vi "Logging Message Loop.vi"(8 "error in (no error)":errorcluster, 10 "Data Queue":refnum<queue>, 11 "Message Queues":T1) -> (0 "error out":errorcluster)   [LabVIEW 2023, in "Logging.lvlib"]
doc: "The message loop subVI to handle messages pertaining to logging data."
uses:
  Logging.lvlib
  support/Message Queue/All Message Queues.ctl
  support/Message Queue/Message Cluster.ctl
  Logging Configuration.ctl
  Logging State.ctl
  support/Message Queue/Enqueue Message (Single).vi
  <vilib>/Utility/error.llb/Error Cluster From Error Code.vi
  <vilib>/ErrorRing/Error Ring.xnode
  support/Message Queue/Message Queue.lvlib
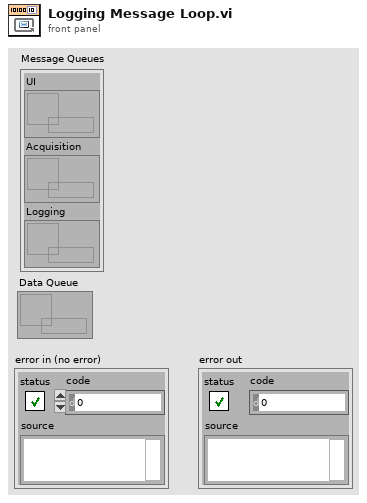
[diagram p1: front panel]
types:
  T1 = typedef "Message Queue.lvlib/All Message Queues.ctl" = cluster{"UI":refnum<queue>, "Acquisition":refnum<queue>, "Logging":refnum<queue>}
  T2 = typedef "Logging.lvlib/Logging Configuration.ctl" = cluster{"Log File Base Path":path, "TDMS File Reference":refnum<k34>}
  T3 = typedef "Logging.lvlib/Logging State.ctl" = enum16{"Idle", "Logging"}
  T4 = enum16{"open", "open or create", "create or replace", "create", "open (read-only)"}
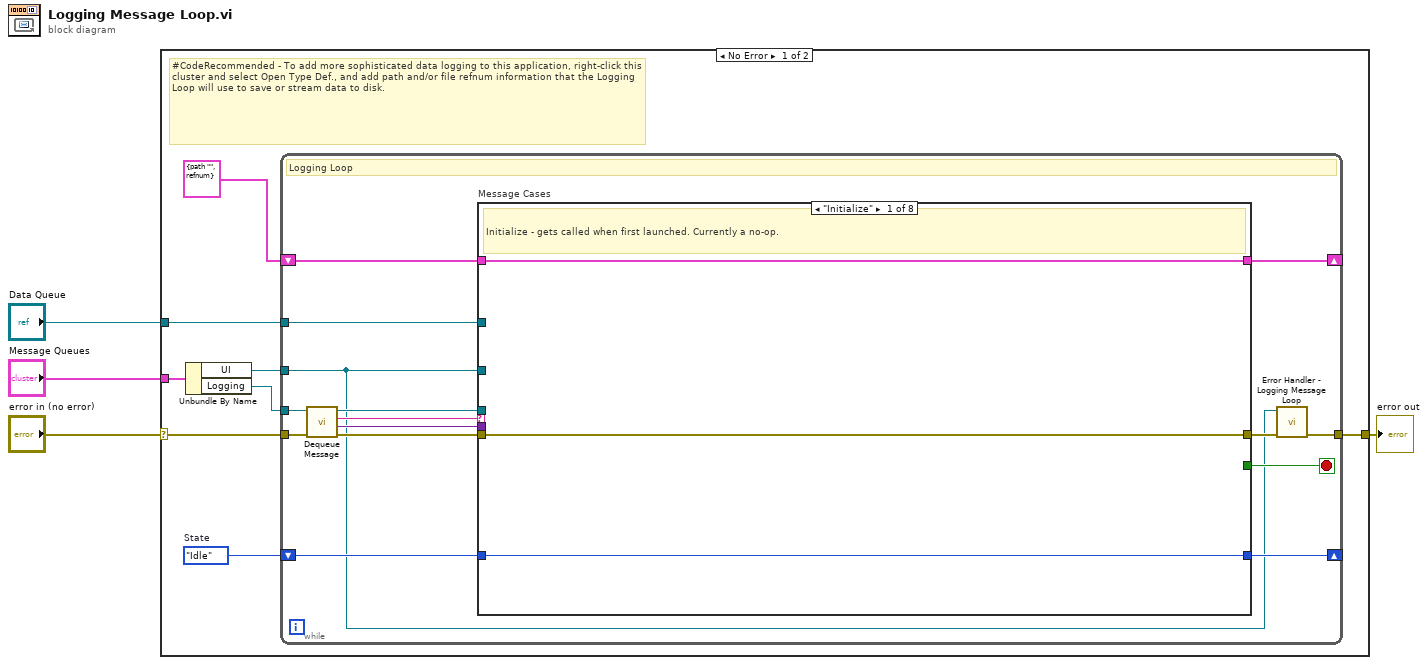
[diagram p0: block diagram]
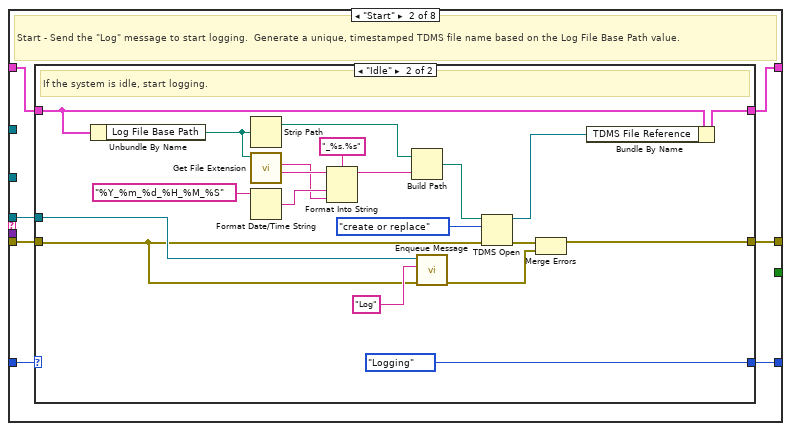
[diagram p2: hidden frame]
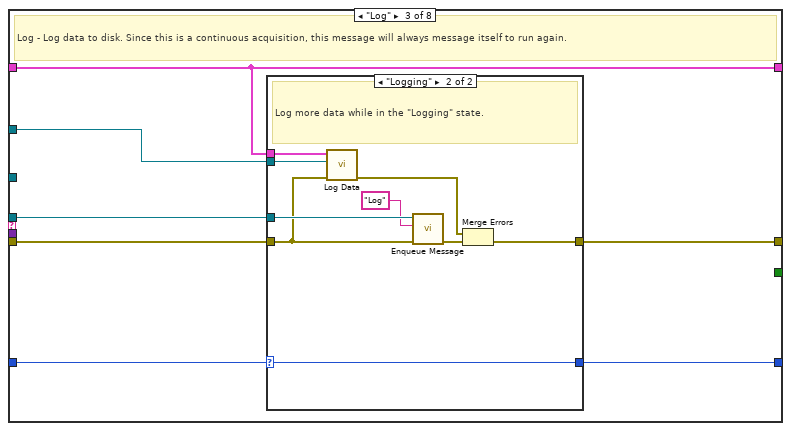
[diagram p4: hidden frame]
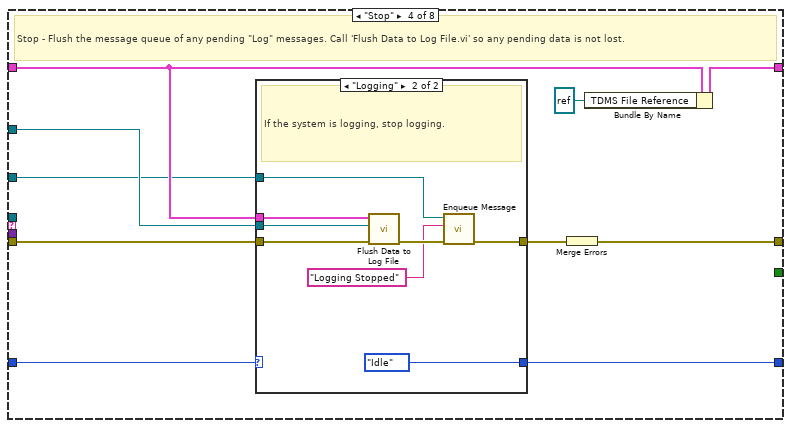
[diagram p6: hidden frame]
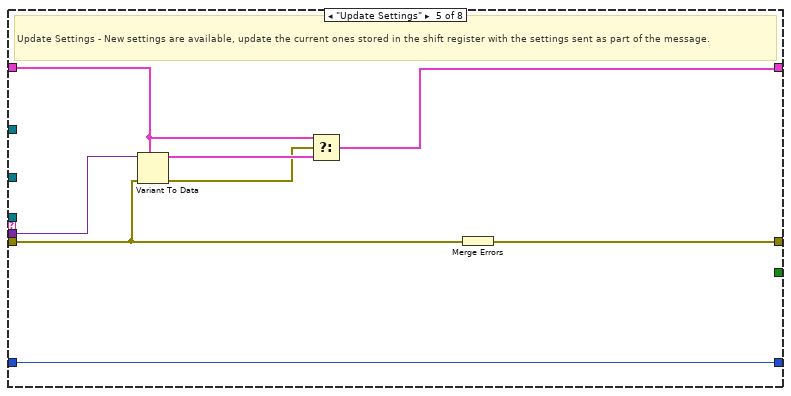
[diagram p8: hidden frame]
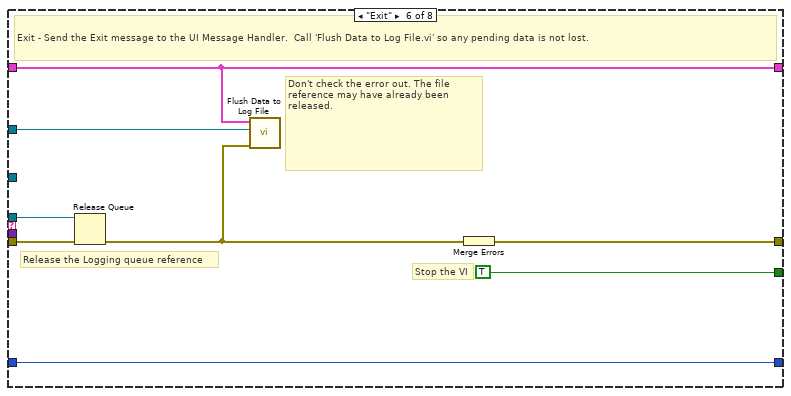
[diagram p9: hidden frame]
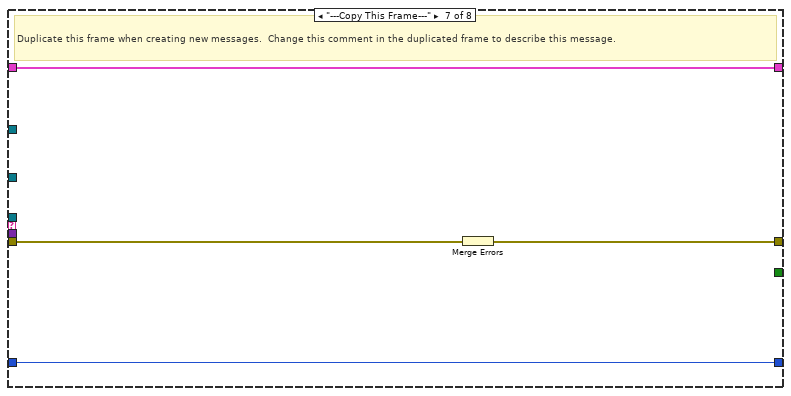
[diagram p10: hidden frame]
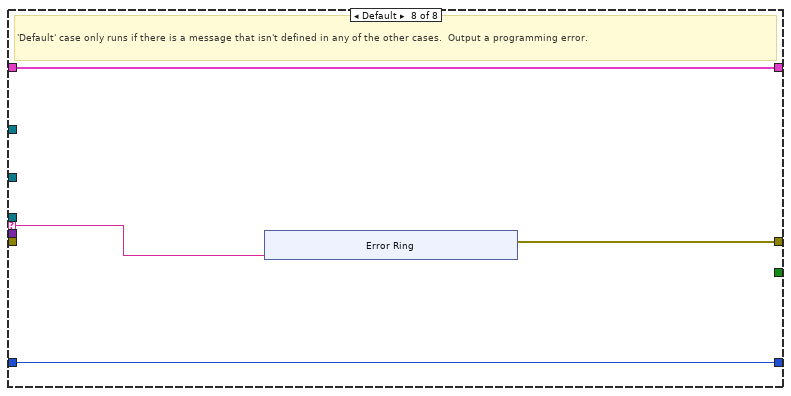
[diagram p11: hidden frame]
diagram:
  n1 = case shown="No Error" "error in (no error)" {
    selector: "error in (no error)" -> [w8 w130]
    tunnel: "Message Queues" -> [w12 _]
    tunnel: [w10 w130] -> w3
    tunnel: "Data Queue" -> [w7 _]
    frame No Error {
      w5 = Logging_State."Idle"  # State
      # "#CodeRecommended - To add more sophisticated data logging to this application, right-click this cluster and select Open Type Def., and add path and/or file refnum information that the Logging Loop will use to save or stream data to disk."
      n2 = Unbundle By Name(w12) -> ("UI"=w6:refnum<queue>, "Logging"=w11:refnum<queue>)
      n3 = while {
        tunnel: w11 -> [w19]
        shift-right: [w26] -> _
        shift-left: T2 {"Log File Base Path"=path "", "TDMS File Reference"=refnum} ("Logging Configuration") -> [w27]
        tunnel: w6 -> [w13]
        tunnel: w7 -> [w18]
        shift-right: [w16] -> _
        shift-left: w5 -> [w17]
        tunnel: w8 -> [w24]
        tunnel: [w15] -> w10
        stop <- w25 stop-if-true
        # "Logging Loop"
        n4 = call "Dequeue Message.vi"("error in (no error)"=w24, "Message Queue"=w19) -> ("error out"=w23:errorcluster, "Message Data"=w21:variant, "Message"=w22:string, "dup Message Queue"=w20:refnum<queue>)  [unwired: 6 in]
        n5 = case "Message Cases" shown="\"Initialize\"" w22 {
          selector: w22 -> [_ _ _ _ _ _ _ w119]
          tunnel: w20 -> [_ w36 w66 _ _ w111 _ _]
          tunnel: w23 -> [w29 w35 w64 w82 w100 w112 w118 _]
          tunnel: [w29 w37 w67 w88 w106 w113 w116 w120] -> w14
          tunnel: w27 -> [w30 w34 w63 w83 w104 w109 w117 w122]
          tunnel: [w30 w33 w63 w86 w101 w109 w117 w122] -> w26
          tunnel: [_ _ _ _ _ TRUE _ _] -> w25
          tunnel: w21 -> [_ _ _ _ w105 _ _ _]
          tunnel: w13 -> [_ _ _ w79 _ _ _ _]
          tunnel: w18 -> [_ _ w65 w84 _ w108 _ _]
          tunnel: w17 -> [w28 w32 w62 w81 w99 w107 w115 w121]
          tunnel: [w28 w31 w61 w80 w99 w107 w115 w121] -> w16
          frame "Initialize" {
            # "Initialize - gets called when first launched. Currently a no-op."
          }
          frame "Start" {
            # "Start - Send the \"Log\" message to start logging.  Generate a unique, timestamped TDMS file name based on the Log File Base Path value."
            n6 = case shown="\"Idle\"" w32 {
              selector: w32 -> [w39 _]
              tunnel: [w38 w42] -> w37
              tunnel: w36 -> [_ w43]
              tunnel: w35 -> [w38 w41]
              tunnel: w34 -> [w40 w44]
              tunnel: [w40 w46] -> w33
              tunnel: [w39 Logging_State."Logging" ("State")] -> w31
              frame "Logging" {
                # "The system is already logging. Ignore the \"Start\" message."
              }
              frame "Idle" {
                # "If the system is idle, start logging."
                n7 = Unbundle By Name(w44) -> ("Log File Base Path"=w59:path)
                n8 = Strip Path(path=w59) -> (stripped path=w56:path)  [unwired: 1 out]
                n9 = call <vilib>:"Get File Extension.vi"("file"=w59) -> ("filename without extension"=w57:string, "lowercase file extension"=w53:string)  [unwired: 6 in, 3 out]
                n10 = Format Date/Time String(time format string (%c)="%Y_%m_%d_%H_%M_%S") -> (date/time string=w54:string)  [unwired: 2 in]
                n11 = Format Into String(format string="_%s.%s", initial string=w57, w54, w53) -> (resulting string=w52:string)  [unwired: 1 in, 1 out]
                n12 = Build Path(base path=w56, name or relative path=w52) -> (appended path=w51:path)
                n13 = call-poly "Enqueue Message.vi"("error in (no error)"=w41, "Message"="Log", "Message Queue"=w43) -> ("error out"=w49:errorcluster)  [unwired: 7 in, 1 out]
                n14 = TDMS Open(8:w41, 10:T4."create or replace" ("operation (0:open)"), 11:w51) -> (0:w50:errorcluster, 3:w47:refnum<k34>)  [unwired: 4 in]
                n15 = Merge Errors(w50, w49) -> (w42:errorcluster)
                n16 = Bundle By Name(cluster=w44, "TDMS File Reference"=w47) -> (w46:T2)
              }
            }
          }
          frame "Log" {
            # "Log - Log data to disk. Since this is a continuous acquisition, this message will always message itself to run again."
            n17 = case shown="\"Logging\"" w62 {
              selector: w62 -> [w69 w71]
              tunnel: [w68 w78] -> w67
              tunnel: w66 -> [_ w76]
              tunnel: w65 -> [_ w75]
              tunnel: w64 -> [w68 w70]
              tunnel: w63 -> [_ w72]
              tunnel: [w69 w71] -> w61
              frame "Idle" {
                # "Ignore \"Log\" messages when the logging is idle."
              }
              frame "Logging" {
                # "Log more data while in the \"Logging\" state."
                n18 = call "Log Data.vi"("error in (no error)"=w70, "Data Queue"=w75, "Logging Configuration"=w72) -> ("error out"=w74:errorcluster)  [unwired: 8 in]
                n19 = call-poly "Enqueue Message.vi"("error in (no error)"=w70, "Message"="Log", "Message Queue"=w76) -> ("error out"=w77:errorcluster)  [unwired: 7 in, 1 out]
                n20 = Merge Errors(w74, w77) -> (w78:errorcluster)
              }
            }
          }
          frame "Stop" {
            # "Stop - Flush the message queue of any pending \"Log\" messages. Call 'Flush Data to Log File.vi' so any pending data is not lost."
            n21 = case shown="\"Logging\"" w81 {
              selector: w81 -> [w89 _]
              tunnel: [w90 w93] -> w87
              tunnel: w84 -> [_ w97]
              tunnel: w83 -> [_ w96]
              tunnel: w82 -> [w90 w95]
              tunnel: [w89 Logging_State."Idle" ("State")] -> w80
              tunnel: w79 -> [_ w92]
              frame "Idle" {
                # "The system is already idle. Ignore the \"Stop\" message."
              }
              frame "Logging" {
                # "If the system is logging, stop logging."
                n22 = call "Flush Data to Log File.vi"("error in (no error)"=w95, "Data Queue"=w97, "Logging Configuration"=w96) -> ("error out"=w98:errorcluster)  [unwired: 8 in]
                n23 = call-poly "Enqueue Message.vi"("error in (no error)"=w98, "Message"="Logging Stopped", "Message Queue"=w92) -> ("error out"=w93:errorcluster)  [unwired: 7 in, 1 out]
              }
            }
            n24 = Merge Errors(w87) -> (w88:errorcluster)
            n25 = Bundle By Name(cluster=w83, "TDMS File Reference"=refnum<k34> refnum) -> (w86:T2)
          }
          frame "Update Settings" {
            # "Update Settings - New settings are available, update the current ones stored in the shift register with the settings sent as part of the message."
            n26 = Variant To Data(error in=w100, type=w104, Variant=w105) -> (data=w103:T2, error out=w102:errorcluster)
            n27 = Select(t=w104, s=w102, f=w103) -> (s? t:f=w101:T2)
            n28 = Merge Errors(w100) -> (w106:errorcluster)
          }
          frame "Exit" {
            # "Don't check the error out. The file reference may have already been released."
            # "Release the Logging queue reference"
            # "Stop the VI"
            # "Exit - Send the Exit message to the UI Message Handler.  Call 'Flush Data to Log File.vi' so any pending data is not lost."
            n29 = Release Queue(queue=w111, error in (no error)=w112) -> (error out=w110:errorcluster)  [unwired: 1 in, 2 out]
            n30 = call "Flush Data to Log File.vi"("error in (no error)"=w110, "Data Queue"=w108, "Logging Configuration"=w109) -> ()  [unwired: 8 in, 1 out]
            n31 = Merge Errors(w110) -> (w113:errorcluster)
          }
          frame "---Copy This Frame---" {
            # "Duplicate this frame when creating new messages.  Change this comment in the duplicated frame to describe this message."
            n32 = Merge Errors(w118) -> (w116:errorcluster)
          }
          frame Default {
            # "'Default' case only runs if there is a message that isn't defined in any of the other cases.  Output a programming error."
            n33 = xnode "Error Ring"("parameter 0"=w119) -> ("error out"=w120:errorcluster)
          }
        }
        n34 = call "Error Handler - Logging Message Loop.vi"("error in (no error)"=w14, "Message Queue"=w13) -> ("dup error in"=w15:errorcluster)  [unwired: 8 in, 1 out]
      }
    }
    frame Error {
    }
  }
  "error out" <- w3
